vi "_checkForValidToken.vi"(8 "error in (no error)":errorcluster, 9 "String":string, 10 "Token Type":T1=enum."Other", 11 "tJSONParser in":refnum<class "tJSONParser.lvclass">) -> (0 "error out":errorcluster, 3 "tJSONParser out":refnum<class "tJSONParser.lvclass">)   [LabVIEW 2013, in "JSON.lvlib" / "tJSONParser.lvclass"]
doc: "Checks number, boolean, and null strings token-by-token for validity."
uses:
  tJSONParser.lvclass
  _tokenType.ctl
  _error.ctl
  <vilib>/regexp/Match Regular Expression.xnode
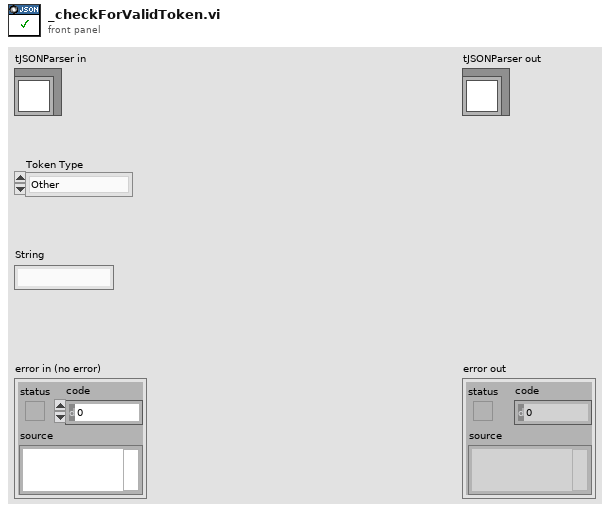
[diagram p1: front panel]
types:
  T1 = typedef "JSON.lvlib/tJSONParser.lvclass/_tokenType.ctl" = enum16{"Object Begin", "Object End", "Array Begin", "Array End", "String Delimeter", "Forward Slash", "Number", "Boolean", "Null", "Object Or Array Separator", "Pair Separator", "End Of File", "Asterisk", "Backward Slash", "Other"}
  T2 = typedef "JSON.lvlib/tJSONParser.lvclass/_error.ctl" = enum16{"Missing Object Open", "Missing Pair Separator", "Missing Object End Or Separator", "Missing Pair String", "Unexpected Token", "Missing Array End Or Separator", "Invalid Escape Sequence", "Unexpected End Of File", "Invalid Unicode", "Unexpected End Of Line", "Invalid Numerical Constant"}
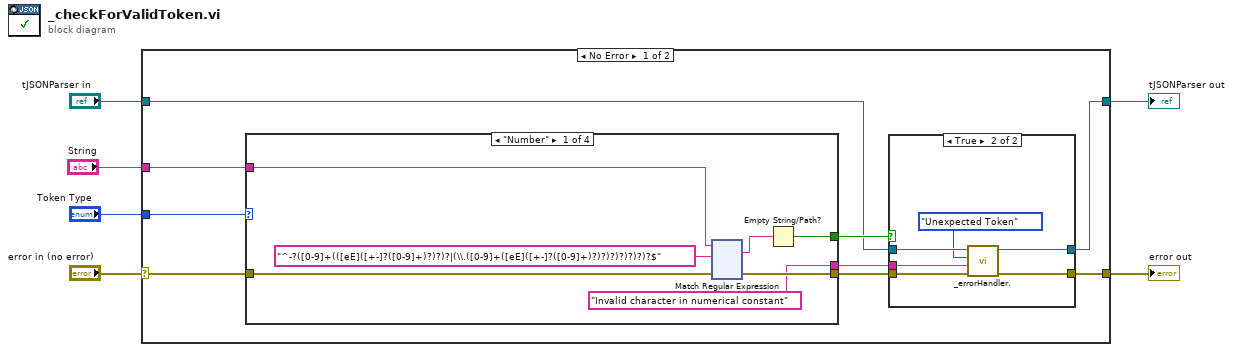
[diagram p0: block diagram]
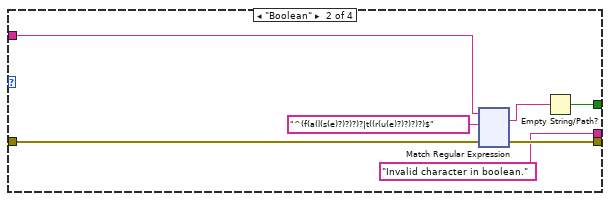
[diagram p3: hidden frame]
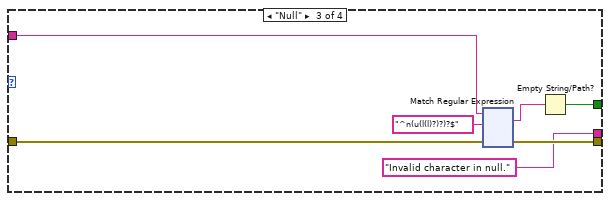
[diagram p4: hidden frame]
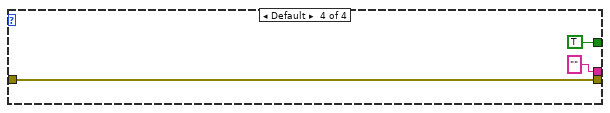
[diagram p5: hidden frame]
diagram:
  n1 = case shown="No Error" "error in (no error)" {
    selector: "error in (no error)" -> [w13 w382]
    tunnel: [w11 w382] -> w5
    tunnel: [w8 w381] -> w3
    tunnel: "tJSONParser in" -> [w9 w381]
    tunnel: "Token Type" -> [w15 _]
    tunnel: "String" -> [w14 _]
    frame No Error {
      n2 = case shown="\"Number\"" w15 {
        tunnel: w14 -> [w28 w145 w262 _]
        tunnel: w13 -> [w30 w147 w264 w380]
        tunnel: [w29 w146 w263 w380] -> w12
        tunnel: [w26 w144 w261 TRUE] -> w10
        tunnel: ["Invalid character in numerical constant" "Invalid character in boolean." "Invalid character in null." ""] -> w7
        frame "Number" {
          n3 = xnode "Match Regular Expression"("input string"=w28, "regular expression"="^-?([0-9]+(([eE]([+-]?([0-9]+)?)?)?|(\\.([0-9]+([eE]([+-]?([0-9]+)?)?)?)?)?)?)?$", "error in"=w30) -> ("whole match"=w27:string, "error out"=w29:errorcluster)  [unwired: 3 in, 3 out]
          n4 = Empty String/Path?(string/path=w27) -> (empty?=w26:bool)
        }
        frame "Boolean" {
          n5 = xnode "Match Regular Expression"("input string"=w145, "regular expression"="^(f(a(l(s(e)?)?)?)?|t((r(u(e)?)?)?)?)$", "error in"=w147) -> ("whole match"=w148:string, "error out"=w146:errorcluster)  [unwired: 3 in, 3 out]
          n6 = Empty String/Path?(string/path=w148) -> (empty?=w144:bool)
        }
        frame "Null" {
          n7 = xnode "Match Regular Expression"("input string"=w262, "regular expression"="^n(u(l(l)?)?)?$", "error in"=w264) -> ("whole match"=w265:string, "error out"=w263:errorcluster)  [unwired: 3 in, 3 out]
          n8 = Empty String/Path?(string/path=w265) -> (empty?=w261:bool)
        }
        frame Default {
        }
      }
      n9 = case shown="True" w10 {
        tunnel: w12 -> [w17 w23]
        tunnel: [w17 w22] -> w11
        tunnel: w9 -> [w16 w21]
        tunnel: [w16 w20] -> w8
        tunnel: w7 -> [_ w18]
        frame False {
        }
        frame True {
          n10 = call "_errorHandler..vi"("error in (no error)"=w23, "Additional Text"=w18, "Error Type"=_error."Unexpected Token", "JSON Parser In"=w21) -> ("error out"=w22:errorcluster, "JSON Parser Out"=w20:refnum<class "tJSONParser.lvclass">)  [unwired: 6 in]
        }
      }
    }
    frame Error {
    }
  }
  "error out" <- w5
  "tJSONParser out" <- w3
